vi "CP_Cmd_Setting.vi"(7 "CP Setting":dbl[](array[numeric])=[0.0, 23.75, 24.5, 25.25, 26.0, 26.75, 27.5, 28.25, 29.0, 29.75, 30.5, 31.25, 32.0, 32.75, 33.5, 34.25, 35.0, 35.75, 36.5, 37.25, 38.0, 38.75, 39.5, 40.25, 41.0, 41.75, 42.5, 43.25, 44.0, 50.0, 55.0], 8 "error in (no error)":errorcluster, 11 "Input":dbl) -> (0 "error out":errorcluster, 2 "CP Voltage":string, 3 "Send Cmd":string, 4 "Array":bool[](array[boolean]))   [LabVIEW 2012]
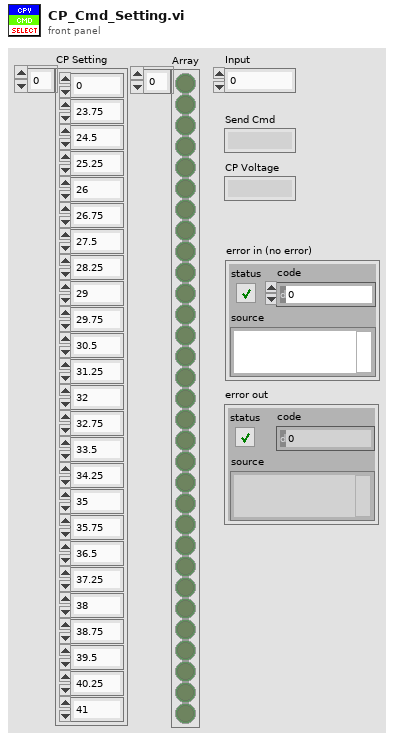
[diagram p1: front panel]
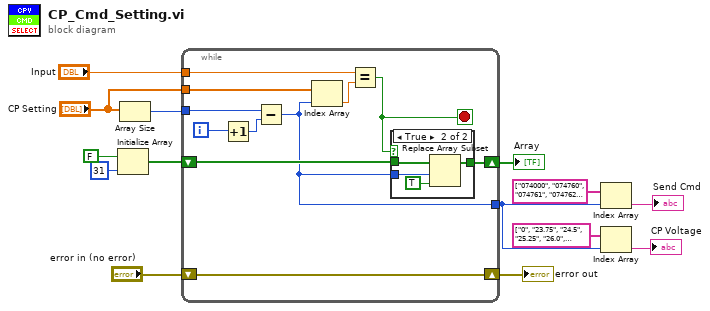
[diagram p0: block diagram]
diagram:
  n1 = Initialize Array(FALSE, 31 ("dimension size")) -> (w11:bool[])
  n2 = Array Size(array="CP Setting") -> (size(s)=w14:i32)
  n3 = while {
    tunnel: w14 -> [w23]
    tunnel: "CP Setting" -> [w24]
    tunnel: "Input" -> [w20]
    shift-right: [w18] -> w8
    shift-left: w11 -> [w19]
    tunnel: [w16] -> w5
    shift-right: [w15] -> w1
    shift-left: "error in (no error)" -> [w15]
    i -> [w25]
    stop <- w17 stop-if-true
    n4 = Increment(x=w25) -> (x+1=w22:i32)
    n5 = Subtract(x=w23, y=w22) -> (x-y=w16:i32)
    n6 = Index Array(array=w24, index=w16) -> (element=w21:dbl)
    n7 = Equal?(x=w20, y=w21) -> (x = y?=w17:bool)
    n8 = case shown="True" w17 {
      tunnel: w19 -> [w26 w30]
      tunnel: w16 -> [_ w29]
      tunnel: [w26 w27] -> w18
      frame False {
      }
      frame True {
        n9 = Replace Array Subset(array=w30, new element=TRUE ("new element/subarray"), index=w29) -> (w27:bool[])
      }
    }
  }
  "Array" <- w8
  "error out" <- w1
  n10 = Index Array(array=string[] ["074000", "074760", "074761", "074762", "074763", "074764", "074765", "074766", "074767", "074768", "074769", "07476A", "07476B", "07476C", "07476D", "07476E", "07476F", "074770", "074771", "074772", "074773", "074774", "074775", "074776", "074777", "074778", "074779", "07477A", "07477B", "07477C", "07477D"], index=w5) -> (element=→"Send Cmd":string)
  n11 = Index Array(array=string[] ["0", "23.75", "24.5", "25.25", "26.0", "26.75", "27.5", "28.25", "29.0", "29.75", "30.5", "31.25", "32.0", "32.75", "33.5", "34.25", "35.0", "35.75", "36.5", "37.25", "38.0", "38.75", "39.5", "40.25", "41.0", "41.75", "42.5", "43.25", "44.0", "50.0", "55.0"], index=w5) -> (element=→"CP Voltage":string)
